vi "GetMimeType.vi"(3 "Extension":string) -> (1 "mimetype":string)   [LabVIEW 2016]
doc: "Returns the mime type"
panel:
  out "mimetype":string[](array[string])
  out "extension":string[](array[string])
  in  "String":string="acx\napplication/internet-property-stream\nai\napplication/postscript\naif\naudio/x-aiff\naifc\naudio/x-aiff\naiff\naudio/x-aiff\nasf\nvideo/x-ms-asf\nasr\nvideo/x-ms-asf\nasx\nvideo/x-ms-asf\nau\naudio/basic\navi\nvideo/x-msvideo\naxs\napplication/olescript\nbas\ntext/plain\nbcpio\napplication/x-bcpio\nbin\napplication/octet-stream\nbmp\nimage/bmp\nc\ntext/plain\ncat\napplication/vnd.ms-pkiseccat\ncdf\napplication/x-cdf\ncer\napplication/x-x509-ca-cert\nclass\napplication/octet-stream\nclp\napplication/x-msclip\ncmx\nimage/x-cmx\ncod\nimage/cis-cod\ncpio\napplication/x-cpio\ncrd\napplication/x-mscardfile\ncrl\napplication/pkix-crl\ncrt\napplication/x-x509-ca-cert\ncsh\napplication/x-csh\ncss\ntext/css\ndcr\napplication/x-director\nder\napplication/x-x509-ca-cert\ndir\napplication/x-director\ndll\napplication/x-msdownload\ndms\napplication/octet-stream\ndoc\napplication/msword\ndot\napplication/msword\ndvi\napplication/x-dvi\ndxr\napplication/x-director\neps\napplication/postscript\netx\ntext/x-setext\nevy\napplication/envoy\nexe\napplication/octet-stream\nfif\napplication/fractals\nflr\nx-world/x-vrml\nflv\nvideo/x-flv\ngif\nimage/gif\ngtar\napplication/x-gtar\ngz\napplication/x-gzip\nh\ntext/plain\nhdf\napplication/x-hdf\nhlp\napplication/winhlp\nhqx\napplication/mac-binhex40\nhta\napplication/hta\nhtc\ntext/x-component\nhtm\ntext/html\nhtml\ntext/html\nhtt\ntext/webviewhtml\nico\nimage/x-icon\nief\nimage/ief\niii\napplication/x-iphone\nins\napplication/x-internet-signup\nisp\napplication/x-internet-signup\njfif\nimage/pipeg\njpe\nimage/jpeg\njpeg\nimage/jpeg\njpg\nimage/jpeg\njs\napplication/x-javascript\nlatex\napplication/x-latex\nlha\napplication/octet-stream\nlsf\nvideo/x-la-asf\nlsx\nvideo/x-la-asf\nlzh\napplication/octet-stream\nm13\napplication/x-msmediaview\nm14\napplication/x-msmediaview\nm3u\naudio/x-mpegurl\nman\napplication/x-troff-man\nmdb\napplication/x-msaccess\nme\napplication/x-troff-me\nmht\nmessage/rfc822\nmhtml\nmessage/rfc822\nmid\naudio/mid\nmny\napplication/x-msmoney\nmov\nvideo/quicktime\nmovie\nvideo/x-sgi-movie\nmp2\nvideo/mpeg\nmp3\naudio/mpeg\nmp4\nvideo/mpeg\nmpa\nvideo/mpeg\nmpe\nvideo/mpeg\nmpeg\nvideo/mpeg\nmpg\nvideo/mpeg\nmpp\napplication/vnd.ms-project\nmpv2\nvideo/mpeg\nms\napplication/x-troff-ms\nmvb\napplication/x-msmediaview\nnws\nmessage/rfc822\noda\napplication/oda\np10\napplication/pkcs10\np12\napplication/x-pkcs12\np7b\napplication/x-pkcs7-certificates\np7c\napplication/x-pkcs7-mime\np7m\napplication/x-pkcs7-mime\np7r\napplication/x-pkcs7-certreqresp\np7s\napplication/x-pkcs7-signature\npbm\nimage/x-portable-bitmap\npdf\napplication/pdf\npfx\napplication/x-pkcs12\npgm\nimage/x-portable-graymap\npko\napplication/ynd.ms-pkipko\npma\napplication/x-perfmon\npmc\napplication/x-perfmon\npml\napplication/x-perfmon\npmr\napplication/x-perfmon\npmw\napplication/x-perfmon\npng\nimage/png\npnm\nimage/x-portable-anymap\npot,\napplication/vnd.ms-powerpoint\nppm\nimage/x-portable-pixmap\npps\napplication/vnd.ms-powerpoint\nppt\napplication/vnd.ms-powerpoint\nprf\napplication/pics-rules\nps\napplication/postscript\npub\napplication/x-mspublisher\nqt\nvideo/quicktime\nra\naudio/x-pn-realaudio\nram\naudio/x-pn-realaudio\nras\nimage/x-cmu-raster\nrgb\nimage/x-rgb\nrmi\naudio/mid\nroff\napplication/x-troff\nrtf\napplication/rtf\nrtx\ntext/richtext\nscd\napplication/x-msschedule\nsct\ntext/scriptlet\nsetpay\napplication/set-payment-initiation\nsetreg\napplication/set-registration-initiation\nsh\napplication/x-sh\nshar\napplication/x-shar\nsit\napplication/x-stuffit\nsnd\naudio/basic\nspc\napplication/x-pkcs7-certificates\nspl\napplication/futuresplash\nsrc\napplication/x-wais-source\nsst\napplication/vnd.ms-pkicertstore\nstl\napplication/vnd.ms-pkistl\nstm\ntext/html\nsvg\nimage/svg+xml\nsv4cpio\napplication/x-sv4cpio\nsv4crc\napplication/x-sv4crc\nswf\napplication/x-shockwave-flash\nt\napplication/x-troff\ntar\napplication/x-tar\ntcl\napplication/x-tcl\ntex\napplication/x-tex\ntexi\napplication/x-texinfo\ntexinfo\napplication/x-texinfo\ntgz\napplication/x-compressed\ntif\nimage/tiff\ntiff\nimage/tiff\ntr\napplication/x-troff\ntrm\napplication/x-msterminal\ntsv\ntext/tab-separated-values\ntxt\ntext/plain\nuls\ntext/iuls\nustar\napplication/x-ustar\nvcf\ntext/x-vcard\nvrml\nx-world/x-vrml\nwav\naudio/x-wav\nwcm\napplication/vnd.ms-works\nwdb\napplication/vnd.ms-works\nwks\napplication/vnd.ms-works\nwmf\napplication/x-msmetafile\nwmv\nvideo/x-ms-wmv\nwps\napplication/vnd.ms-works\nwri\napplication/x-mswrite\nwrl\nx-world/x-vrml\nwrz\nx-world/x-vrml\nxaf\nx-world/x-vrml\nxbm\nimage/x-xbitmap\nxla\napplication/vnd.ms-excel\nxlc\napplication/vnd.ms-excel\nxlm\napplication/vnd.ms-excel\nxls\napplication/vnd.ms-excel\nxlt\napplication/vnd.ms-excel\nxlw\napplication/vnd.ms-excel\nxml\ntext/xml\nxof\nx-world/x-vrml\nxpm\nimage/x-xpixmap\nxwd\nimage/x-xwindowdump\nz\napplication/x-compress\nzip\napplication/zip\n"
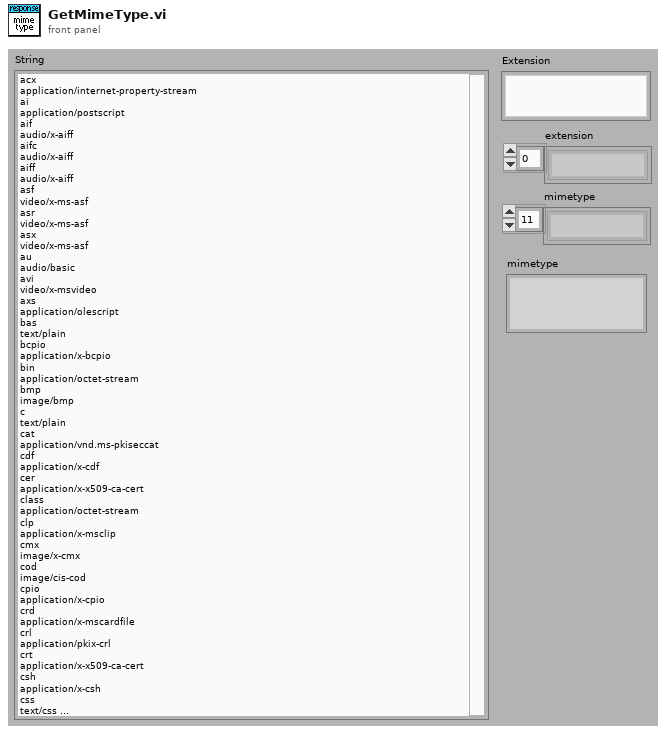
[diagram p1: front panel]
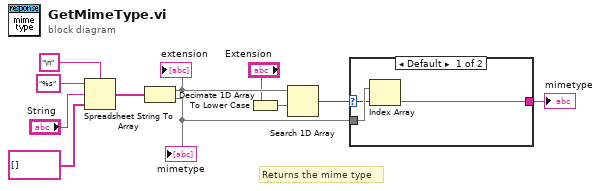
[diagram p0: block diagram]
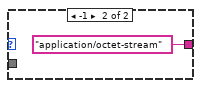
[diagram p2: hidden frame]
diagram:
  # "Returns the mime type"
  n1 = Spreadsheet String To Array(delimiter (Tab)="\n", format string="%s", spreadsheet string="String", array type (2D Dbl)=string[] [] ("extension")) -> (array=w7:string[])
  n2 = Decimate 1D Array(w7) -> (w6:string[], w2:string[])
  "extension" <- w6
  "mimetype" <- w2
  n3 = To Lower Case(string="Extension") -> (all lower case string=w1:string)
  n4 = Search 1D Array(1D array=w6, element=w1) -> (index of element=w4:i32)  [unwired: 1 out]
  n5 = case shown="Default" w4 {
    selector: w4 -> [w13 _]
    tunnel: [w12 "application/octet-stream" ("String")] -> w3
    tunnel: w2 -> [w14 _]
    frame Default {
      n6 = Index Array(array=w14, index=w13) -> (element=w12:string)
    }
    frame -1 {
    }
  }
  "mimetype" <- w3
